vi "Initialize.vi"(8 "error in (no error)":errorcluster, 11 "GSdevice in":refnum<class "GSdevice.lvclass">) -> (0 "error out":errorcluster, 3 "GSdevice out":refnum<class "GSdevice.lvclass">)   [LabVIEW 2018, in "GSdevice.lvclass"]
uses:
  GSdevice.lvclass
  Device/Device.lvclass
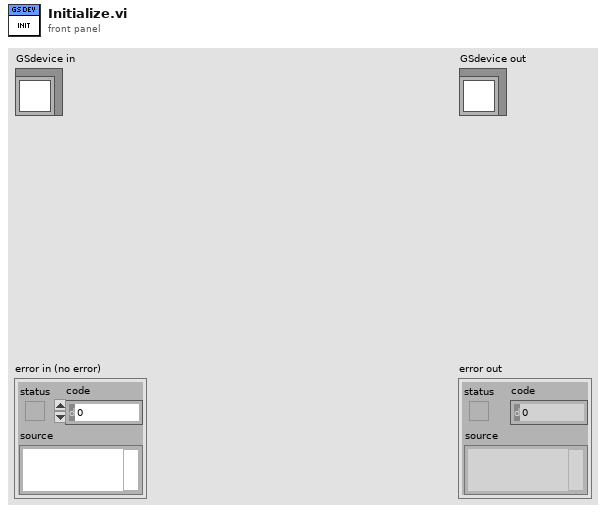
[diagram p1: front panel]
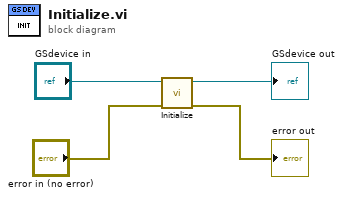
[diagram p0: block diagram]
diagram:
  n1 = call-parent "Initialize.vi"("error in (no error)"="error in (no error)", "Device in"="GSdevice in") -> ("error out"=→"error out":errorcluster, "Device out"=→"GSdevice out":refnum<class "GSdevice.lvclass">)  [unwired: 8 in]
